vi "Robot Web Client.vi"() -> ()   [LabVIEW 2015]
uses:
  <vilib>/httpClient/POSTBuffer.vi
  <vilib>/httpClient/LabVIEWHTTPClient.lvlib
panel:
  out "Current Joint Positions":dbl[](array[numeric]) format="%#_13g"
  out "JointPosition":dbl[](array[numeric])
  in  "MotionEnd":string(combo)="Blend"
  in  "MotionEnd":string(combo)="Blend"
  in  "?":bool
  in  "Accel":i32=100
  in  "Decel":i32=100
  in  "Speed":i32=10
  in  "StraightMotion":bool=TRUE
  in  "SCurveProfile":i32
  in  "Joint 1":dbl
  in  "Joint 3":dbl
  in  "Joint 5":dbl
  in  "Joint 2":dbl
  in  "Joint 4":dbl
  in  "Joint 6":dbl
  out "Joint Move JSON Command":string
  in  "?":bool
  in  "Stop":bool
  in  "?":bool
  out "Cartesian Move JSON Command":string
  in  "Roll":dbl
  in  "Pitch":dbl
  in  "Yaw":dbl
  in  "Z":dbl
  in  "Y":dbl
  in  "X":dbl
  in  "SCurveProfile":i32
  in  "StraightMotion":bool=TRUE
  in  "Speed":i32=10
  in  "Decel":i32=100
  in  "Accel":i32=100
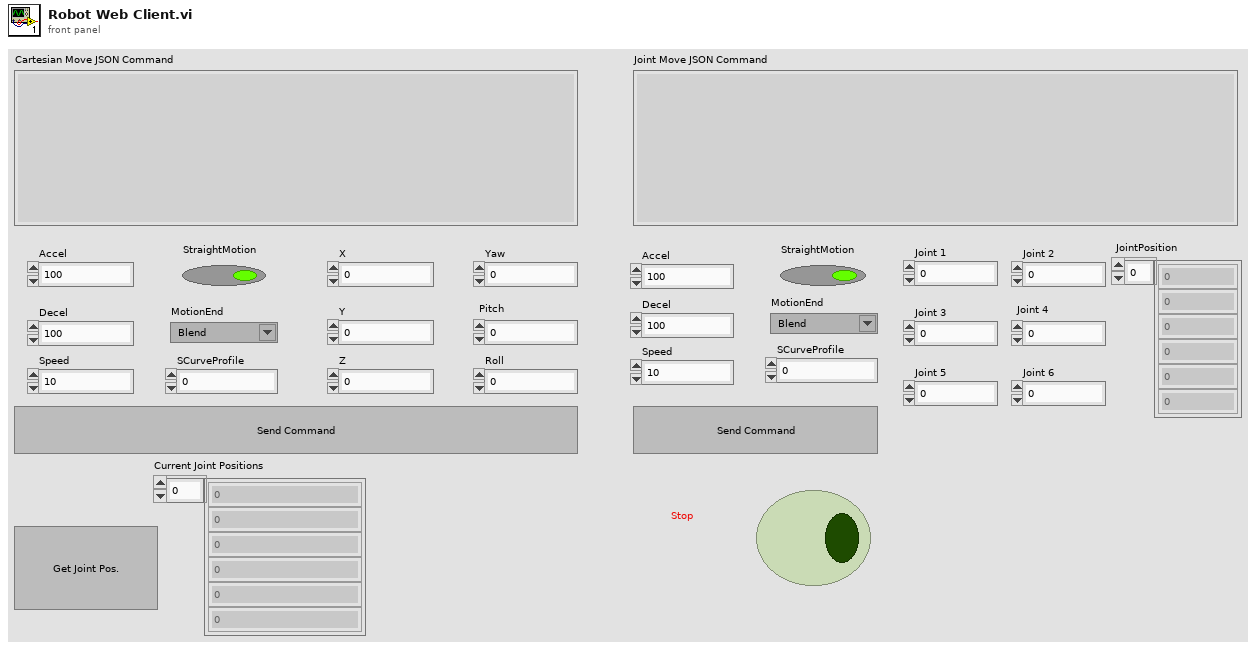
[diagram p1: front panel]
types:
  T1 = typedef "LabVIEWHTTPClient.lvlib/ClientHandle.ctl" = refnum<k1>
  T2 = cluster{"Accel":i32, "Decel":i32, "Speed":i32, "StraightMotion":bool, "MotionEnd":string, "SCurveProfile":i32, "X":dbl, "Y":dbl, "Z":dbl, "Yaw":dbl, "Pitch":dbl, "Roll":dbl}
  T3 = cluster{"Accel":i32, "Decel":i32, "Speed":i32, "StraightMotion":bool, "MotionEnd":string, "SCurveProfile":i32, "JointPosition":dbl[]}
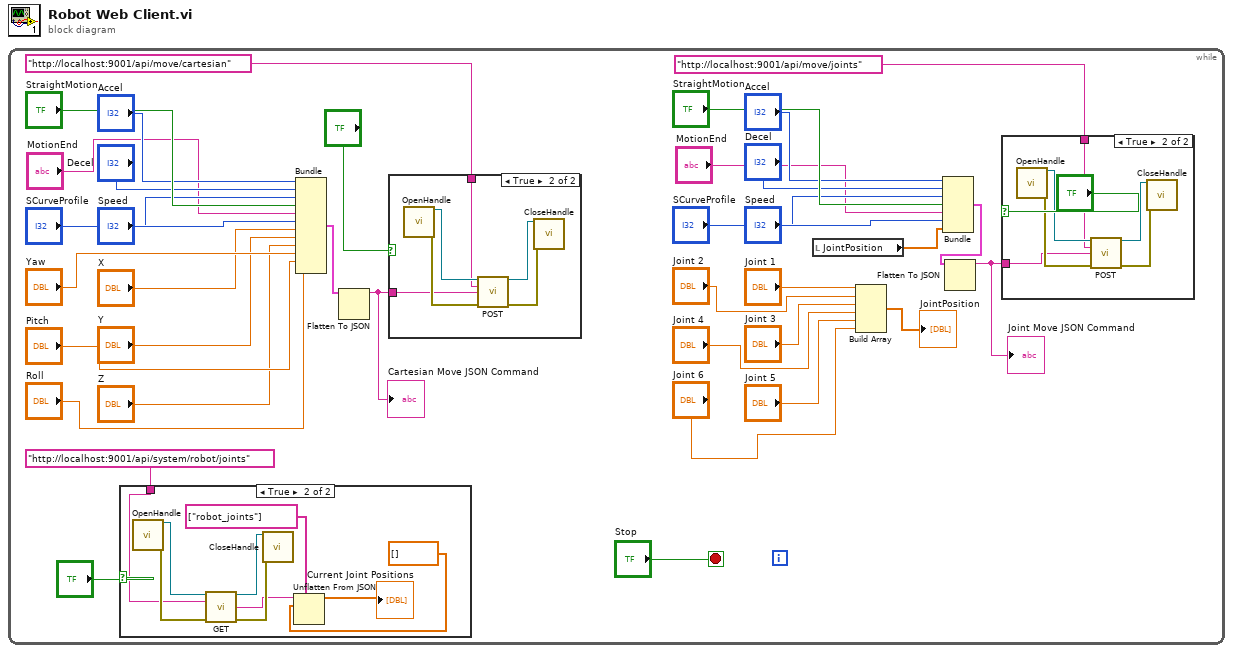
[diagram p0: block diagram]
diagram:
  n1 = while {
    stop <- "Stop" stop-if-true
    n2 = case shown="True" "?" {
      tunnel: "http://localhost:9001/api/system/robot/joints" -> [_ w42]
      frame False {
      }
      frame True {
        n3 = call <vilib>:"OpenHandle.vi"() -> ("client handle out"=w46:T1, "error out"=w45:errorcluster)  [unwired: 14 in]
        n4 = call <vilib>:"GET.vi"("client handle"=w46, "url"=w42, "error in (no error)"=w45) -> ("client handle out"=w44:T1, "body"=w41:string, "error out"=w43:errorcluster)  [unwired: 9 in, 1 out]
        n5 = call <vilib>:"CloseHandle.vi"("client handle"=w44, "error in (no error)"=w43) -> ()  [unwired: 13 in, 1 out]
        n6 = Unflatten From JSON(path=string[] ["robot_joints"], JSON string=w41, type and defaults=dbl[] []) -> (value=→"Current Joint Positions":dbl[])  [unwired: 4 in, 1 out]
      }
    }
    n7 = Bundle("Accel"="Accel", "Decel"="Decel", "Speed"="Speed", "StraightMotion"="StraightMotion", "MotionEnd"="MotionEnd", "SCurveProfile"="SCurveProfile", "X"="X", "Y"="Y", "Z"="Z", "Yaw"="Yaw", "Pitch"="Pitch", "Roll"="Roll") -> (w5:T2)  [unwired: 1 in]
    n8 = Flatten To JSON(anything=w5) -> (JSON string=w6:string)  [unwired: 2 in, 1 out]
    "Cartesian Move JSON Command" <- w6
    n9 = case shown="True" "?" {
      tunnel: "http://localhost:9001/api/move/cartesian" -> [_ w48]
      tunnel: w6 -> [_ w47]
      frame False {
      }
      frame True {
        n10 = call <vilib>:"OpenHandle.vi"() -> ("client handle out"=w50:T1, "error out"=w49:errorcluster)  [unwired: 14 in]
        n11 = call-poly <vilib>:"POST.vi"("client handle"=w50, "url"=w48, "buffer"=w47, "error in (no error)"=w49) -> ("client handle out"=w52:T1, "error out"=w51:errorcluster)  [unwired: 8 in, 2 out]
        n12 = call <vilib>:"CloseHandle.vi"("client handle"=w52, "error in (no error)"=w51) -> ()  [unwired: 13 in, 1 out]
      }
    }
    n13 = local read "JointPosition"() -> (w1:dbl[])
    n14 = Build Array("Joint 1", "Joint 2", "Joint 3", "Joint 4", "Joint 5", "Joint 6") -> (→"JointPosition":dbl[])
    n15 = Bundle("Accel"="Accel", "Decel"="Decel", "Speed"="Speed", "StraightMotion"="StraightMotion", "MotionEnd"="MotionEnd", "SCurveProfile"="SCurveProfile", "JointPosition"=w1) -> (w10:T3)  [unwired: 1 in]
    n16 = Flatten To JSON(anything=w10) -> (JSON string=w9:string)  [unwired: 2 in, 1 out]
    "Joint Move JSON Command" <- w9
    n17 = case shown="True" "?" {
      tunnel: "http://localhost:9001/api/move/joints" -> [_ w54]
      tunnel: w9 -> [_ w53]
      frame False {
      }
      frame True {
        n18 = call <vilib>:"OpenHandle.vi"() -> ("client handle out"=w56:T1, "error out"=w55:errorcluster)  [unwired: 14 in]
        n19 = call-poly <vilib>:"POST.vi"("client handle"=w56, "url"=w54, "buffer"=w53, "error in (no error)"=w55) -> ("client handle out"=w58:T1, "error out"=w57:errorcluster)  [unwired: 8 in, 2 out]
        n20 = call <vilib>:"CloseHandle.vi"("client handle"=w58, "error in (no error)"=w57) -> ()  [unwired: 13 in, 1 out]
      }
    }
  }
